vi "Open Sample Container Dialog.vi"(8 "error in (no error)":errorcluster, 9 "Sample Clipboard Q":refnum<queue>, 10 "Sample Container":T1) -> (0 "error out":errorcluster)   [LabVIEW 2015, in "AMS UI.lvlib" / "AMS Gas.lvclass"]
uses:
  AMS Gas.lvclass
  Controls/Sample Container.ctl
  subs/Sample/Sample.lvclass
panel:
  out "AMS Gas out":refnum<class "AMS Gas.lvclass">
  in  "AMS Gas in":refnum<class "AMS Gas.lvclass">
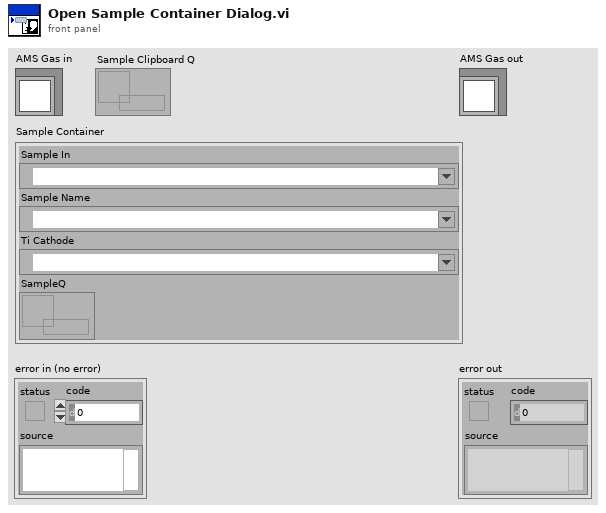
[diagram p1: front panel]
types:
  T1 = typedef "Sample Container.ctl" = cluster{"Sample In":refnum<k21>, "Sample Name":refnum<k21>, "Ti Cathode":refnum<k21>, "SampleQ":refnum<queue>}
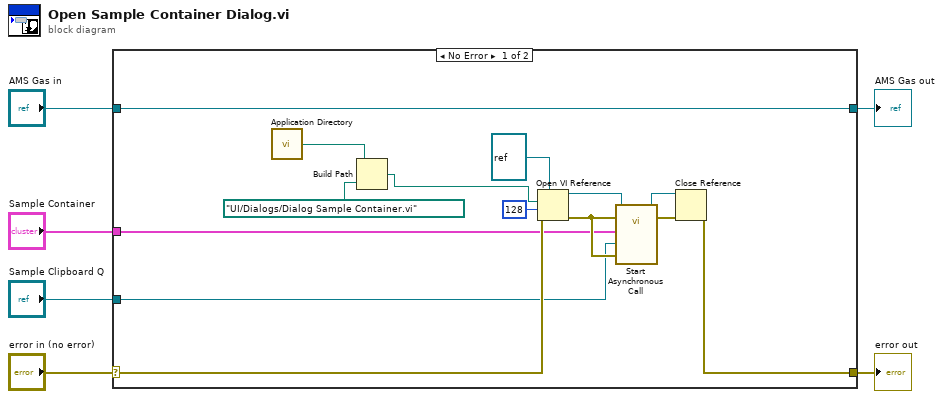
[diagram p0: block diagram]
diagram:
  n1 = case shown="No Error" "error in (no error)" {
    selector: "error in (no error)" -> [w15 w22]
    tunnel: [w13 w22] -> w5
    tunnel: [w20 w21] -> w3
    tunnel: "AMS Gas in" -> [w20 w21]
    tunnel: "Sample Container" -> [w11 _]
    tunnel: "Sample Clipboard Q" -> [w10 _]
    frame No Error {
      n2 = call <vilib>:"Application Directory.vi"() -> ("Application Directory"=w9:path)
      n3 = Build Path(base path=w9, name or relative path=path "UI/Dialogs/Dialog Sample Container.vi" ("vi path")) -> (appended path=w7:path)
      n4 = Open VI Reference(type specifier VI Refnum (for type only)=refnum<vi> refnum, vi path=w7, options=128, error in (no error)=w15) -> (vi reference=w18:refnum<vi>, error out=w17:errorcluster)  [unwired: 2 in]
      n5 = call-by-ref "Start Asynchronous Call"(reference=w18, error in=w17, 8:"error in (no error)"=w17, "Sample Clipboard Q"=w10, "Container"=w11) -> (reference out=w12:refnum<vi>, error out=w14:errorcluster)  [unwired: 7 in, 2 out]
      n6 = Close Reference(reference=w12, error in (no error)=w14) -> (error out=w13:errorcluster)
    }
    frame Error {
    }
  }
  "error out" <- w5
  "AMS Gas out" <- w3
